vi "Fetch PV Data.vi"(7 "PV name":string, 8 "error in":errorcluster, 11 "Source in":refnum<class "Source.lvclass">) -> (0 "error out":errorcluster, 1 "PV found?":bool, 2 "PV Data out":refnum<class "PV Data.lvclass">, 3 "Source out":refnum<class "Source.lvclass">)   [LabVIEW 2020, in "PV Access.lvlib" / "PVA Server.lvlib" / "Source.lvclass"]
uses:
  Source.lvclass
  PV Data/PV Data/PV Data.lvclass
  Source.lvclass/Source.ctl
  PV Access.lvlib
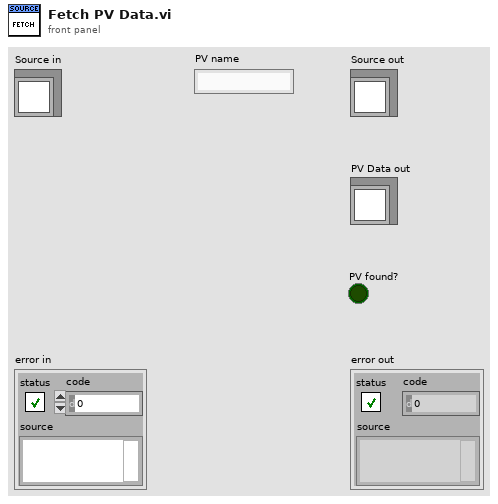
[diagram p1: front panel]
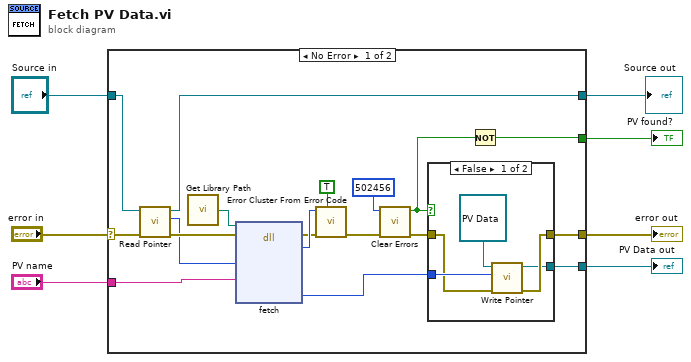
[diagram p0: block diagram]
diagram:
  n1 = case shown="No Error" "error in" {
    selector: "error in" -> [w25 w33]
    tunnel: [w15 w33] -> w6
    tunnel: [w21 w32] -> w2
    tunnel: "PV name" -> [w20 _]
    tunnel: [w14 _] -> w4
    tunnel: "Source in" -> [w16 w32]
    tunnel: [w9 _] -> w1
    frame No Error {
      n2 = call-dynamic "Read Pointer.vi"("error in (no error)"=w25, "Pointer Base in"=w16) -> ("error out"=w24:errorcluster, "Pointer"=w22:i64, "Pointer Base out"=w21:refnum<class "Source.lvclass">)  [unwired: 7 in]
      n3 = call "Get Library Path.vi"() -> ("Path"=w23:path)  [unwired: 1 in]
      n4 = dll-call lib="?" fn="fetch"(path in=w23, error in=w24, "source"=w22, "pv_name"=w20) -> (error out=w17:errorcluster, "ret_code"=w18:i32, "value"=w13:i64)  [unwired: 4 in, 1 out]
      n5 = call <vilib>:"Error Cluster From Error Code.vi"("show call chain? (False)"=TRUE, "error in (no error)"=w17, "error code (0)"=w18) -> ("error out"=w12:errorcluster)  [unwired: 6 in]
      n6 = call <vilib>:"Clear Errors.vi"("error in (no error)"=w12, "specific error code to clear (0: all)"=502456) -> ("error out"=w11:errorcluster, "specific error cleared?"=w8:bool)  [unwired: 4 in]
      n7 = case shown="False" w8 {
        tunnel: [w30 w31] -> w15
        tunnel: [w29 _] -> w14
        tunnel: w13 -> [w27 _]
        tunnel: w11 -> [w26 w31]
        frame False {
          n8 = call-dynamic "Write Pointer.vi"("error in (no error)"=w26, "Pointer"=w27, "Pointer Base in"=refnum<class "PV Data.lvclass"> refnum ("PV Access.lvlib:PV Data.lvlib:PV Data.lvclass")) -> ("error out"=w30:errorcluster, "Pointer Base out"=w29:refnum<class "PV Data.lvclass">)  [unwired: 7 in]
        }
        frame True {
        }
      }
      n9 = Not(x=w8) -> (.not. x?=w9:bool)
    }
    frame Error {
    }
  }
  "error out" <- w6
  "PV Data out" <- w4
  "Source out" <- w2
  "PV found?" <- w1
